vi "2011 Vision.vi"() -> ()   [LabVIEW 2013]
doc: "This example shows how to use color threshold, filtering, and particle analysis to locate reflective tape."
uses:
  Gridded Particles.ctl
  <vilib>/vision/NI_Vision_Development_Module.lvlib
panel:
  in  "stop":bool
  out "Annotated":T1(plugin-control)
  out "Threshold":T1(plugin-control)
  out "Original":T1(plugin-control)
  in  "Files":i32(listbox)
  in  "Filter":bool
  out "Columns":T2
  in  "Luma Range":cluster{"Lower value":i32, "Upper value":i32}={"Lower value"=91, "Upper value"=220}
  in  "Sat Range":cluster{"Lower value":i32, "Upper value":i32}={"Lower value"=50, "Upper value"=221}
  in  "Hue Range":cluster{"Lower value":i32, "Upper value":i32}={"Lower value"=234, "Upper value"=14}
  out "Histogram Xs":T3(graph)
  out "Particle Measurements (pixels)":dbl[][](array[numeric])
  in  "Selection Values":T5(array[cluster])=[{"Measurement Parameter"=35, "Range Lower Value"=5.0, "Range Upper Value"=300.0, "Range"=FALSE, "Measurement Type"=FALSE}] {"Measurement Parameter" items=["Center of Mass X", "Center of Mass Y", "First Pixel X", "First Pixel Y", "Bounding Rect Left", "Bounding Rect Top", "Bounding Rect Right", "Bounding Rect Bottom", "Max Feret Diameter Start X", "Max Feret Diameter Start Y", "Max Feret Diameter End X", "Max Feret Diameter End Y", "Max Horiz. Segment Length Left", "Max Horiz. Segment Length Right", "Max Horiz. Segment Length Row", "-", "Bounding Rect Width", "Bounding Rect Height", "Bounding Rect Diagonal", "Perimeter", "Convex Hull Perimeter", "Holes' Perimeter", "Max Feret Diameter", "Equivalent Ellipse Major Axis", "Equivalent Ellipse Minor Axis", "Equivalent Ellipse Minor Axis (Feret)", "Equivalent Rect Long Side", "Equivalent Rect Short Side", "Equivalent Rect Diagonal", "Equivalent Rect Short Side (Feret)", "Average Horiz. Segment Length", "Average Vert. Segment Length", "Hydraulic Radius", "Waddel Disk Diameter", "-", "Area", "Holes' Area", "Particle & Holes' Area", "Convex Hull Area", "Image Area", "-", "Number of Holes", "Number of Horiz. Segments", "Number of Vert. Segments", "-", "Orientation", "Max Feret Diameter Orientation", "-", "% Area/Image Area", "% Area/(Particle & Holes' Area)", "Ratio of Equivalent Ellipse Axes", "Ratio of Equivalent Rect Sides", "-", "Elongation Factor", "Compactness Factor", "Heywood Circularity Factor", "Type Factor", "-", "Sum X", "Sum Y", "Sum XX", "Sum XY", "Sum YY", "Sum XXX", "Sum XXY", "Sum XYY", "Sum YYY", "-", "Moment of Inertia XX", "Moment of Inertia XY", "Moment of Inertia YY", "Moment of Inertia XXX", "Moment of Inertia XXY", "Moment of Inertia XYY", "Moment of Inertia YYY", "Norm. Moment of Inertia XX", "Norm. Moment of Inertia XY", "Norm. Moment of Inertia YY", "Norm. Moment of Inertia XXX", "Norm. Moment of Inertia XXY", "Norm. Moment of Inertia XYY", "Norm. Moment of Inertia YYY", "Hu Moment 1", "Hu Moment 2", "Hu Moment 3", "Hu Moment 4", "Hu Moment 5", "Hu Moment 6", "Hu Moment 7"]}
  out "Particles post filter":i32
  # "1. Run the VI.\nSelect a folder containing images.\nUntil you abort, you can select an image\nin the list to process."
  # "2. Choose a color range to threshold.\nUse Hue, Saturation, and Luminance ranges. (0-255)\nNote that Red hue is near zero and it may be useful\nto reverse upper/lower to wrap around."
  # "3. Optionally filter using size or other measurements."
  # "4. Histogram indicates where poles are most likely found.\nImage is annotated with green squares around poles.\nParticle measurements can be examined further based on\nshape, size, grouping, location, etc. Columns describes\nthe three most likely columns.\n\nUse the toolbar Stop button to abort."
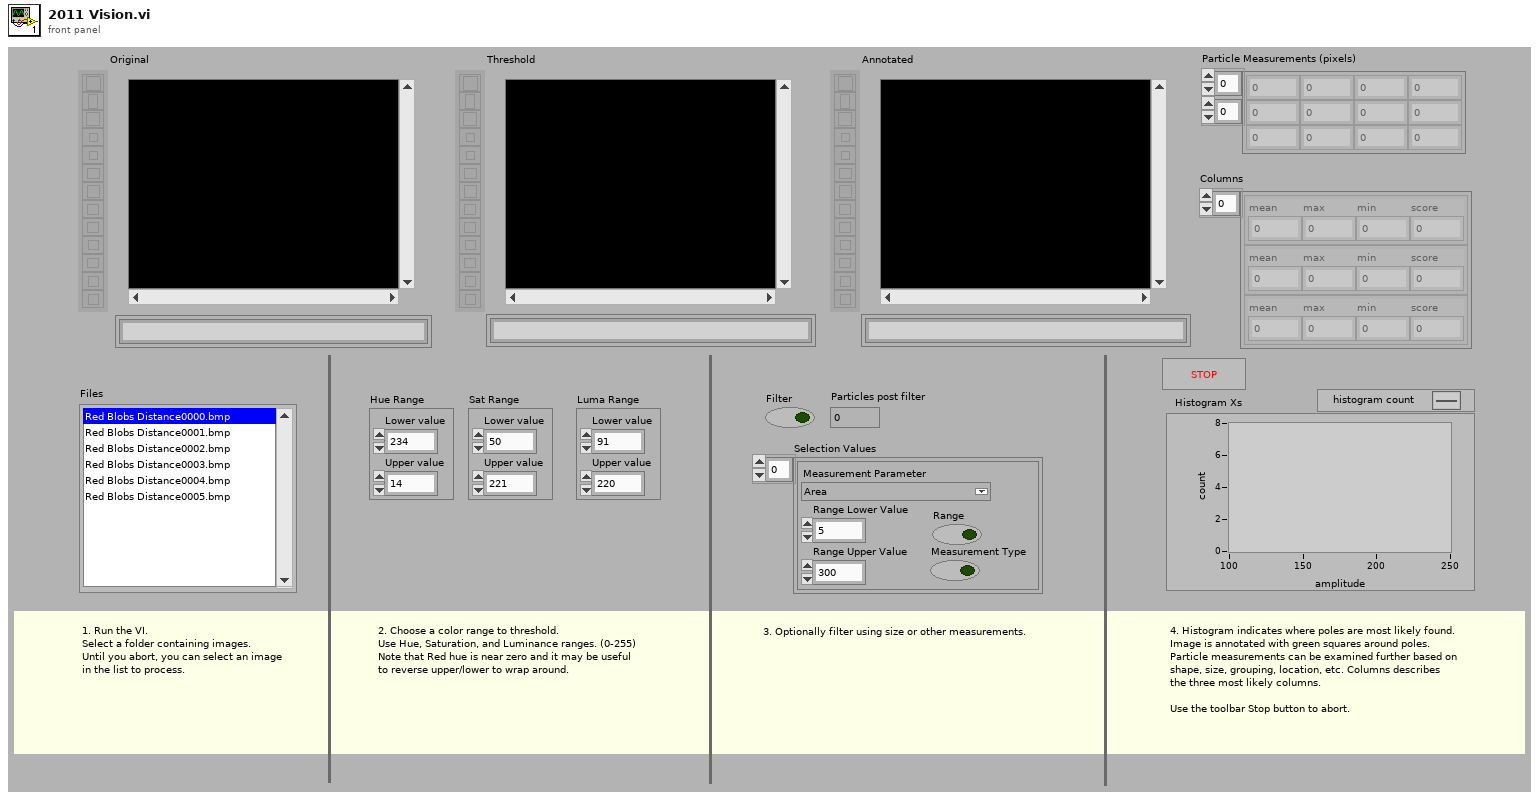
[diagram p1: front panel]
types:
  T1 = typedef "IMAQ Image.ctl" = refnum<image>
  T2 = typedef "Gridded Particles.ctl" = cluster{"mean":dbl, "max":dbl, "min":dbl, "score":dbl}[]
  T3 = cluster{"X Values":dbl[], "Histogram: h(x)":i32[]}
  T4 = typedef "Particle Parameters" = i32
  T5 = cluster{"Measurement Parameter":T4, "Range Lower Value":dbl, "Range Upper Value":dbl, "Range":bool, "Measurement Type":bool}[]
  T6 = typedef "Image Type" = u32
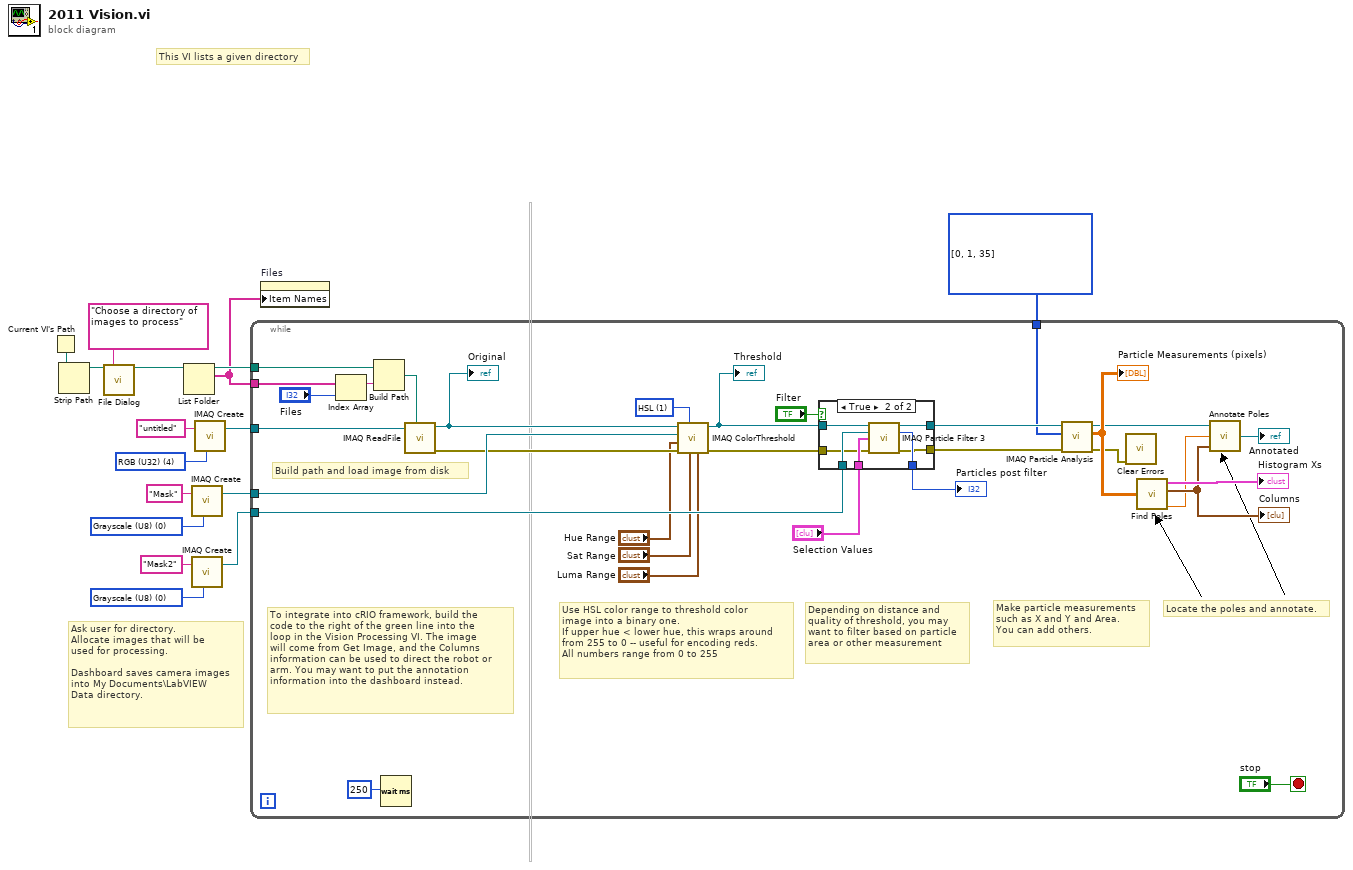
[diagram p0: block diagram]
diagram:
  w4 = T4[] [0, 1, 35] items=["Center of Mass X", "Center of Mass Y", "First Pixel X", "First Pixel Y", "Bounding Rect Left", "Bounding Rect Top", "Bounding Rect Right", "Bounding Rect Bottom", "Max Feret Diameter Start X", "Max Feret Diameter Start Y", "Max Feret Diameter End X", "Max Feret Diameter End Y", "Max Horiz. Segment Length Left", "Max Horiz. Segment Length Right", "Max Horiz. Segment Length Row", "-", "Bounding Rect Width", "Bounding Rect Height", "Bounding Rect Diagonal", "Perimeter", "Convex Hull Perimeter", "Holes' Perimeter", "Max Feret Diameter", "Equivalent Ellipse Major Axis", "Equivalent Ellipse Minor Axis", "Equivalent Ellipse Minor Axis (Feret)", "Equivalent Rect Long Side", "Equivalent Rect Short Side", "Equivalent Rect Diagonal", "Equivalent Rect Short Side (Feret)", "Average Horiz. Segment Length", "Average Vert. Segment Length", "Hydraulic Radius", "Waddel Disk Diameter", "-", "Area", "Holes' Area", "Particle & Holes' Area", "Convex Hull Area", "Image Area", "-", "Number of Holes", "Number of Horiz. Segments", "Number of Vert. Segments", "-", "Orientation", "Max Feret Diameter Orientation", "-", "% Area/Image Area", "% Area/(Particle & Holes' Area)", "Ratio of Equivalent Ellipse Axes", "Ratio of Equivalent Rect Sides", "-", "Elongation Factor", "Compactness Factor", "Heywood Circularity Factor", "Type Factor", "-", "Sum X", "Sum Y", "Sum XX", "Sum XY", "Sum YY", "Sum XXX", "Sum XXY", "Sum XYY", "Sum YYY", "-", "Moment of Inertia XX", "Moment of Inertia XY", "Moment of Inertia YY", "Moment of Inertia XXX", "Moment of Inertia XXY", "Moment of Inertia XYY", "Moment of Inertia YYY", "Norm. Moment of Inertia XX", "Norm. Moment of Inertia XY", "Norm. Moment of Inertia YY", "Norm. Moment of Inertia XXX", "Norm. Moment of Inertia XXY", "Norm. Moment of Inertia XYY", "Norm. Moment of Inertia YYY", "Hu Moment 1", "Hu Moment 2", "Hu Moment 3", "Hu Moment 4", "Hu Moment 5", "Hu Moment 6", "Hu Moment 7"] ("Pixel Measurements")
  w8 = T6 0 items=["Grayscale (U8)", "Grayscale (I16)", "Grayscale (SGL)", "Complex (CSG)", "RGB (U32)", "HSL (U32)", "RGB (U64)", "Grayscale (U16)"] ("Image Type")
  w12 = T6 0 items=["Grayscale (U8)", "Grayscale (I16)", "Grayscale (SGL)", "Complex (CSG)", "RGB (U32)", "HSL (U32)", "RGB (U64)", "Grayscale (U16)"] ("Image Type")
  w15 = T6 4 items=["Grayscale (U8)", "Grayscale (I16)", "Grayscale (SGL)", "Complex (CSG)", "RGB (U32)", "HSL (U32)", "RGB (U64)", "Grayscale (U16)"] ("Image Type")
  # "Ask user for directory.\nAllocate images that will be\nused for processing.\n\nDashboard saves camera images\ninto My Documents\\LabVIEW\nData directory."
  # "This VI lists a given directory"
  n1 = Current VI's Path() -> (path=w1:path)
  n2 = Strip Path(path=w1) -> (stripped path=w2:path)  [unwired: 1 out]
  n3 = call "File Dialog"("start path"=w2, "prompt"="Choose a directory of images to process") -> ("selected path"=w5:path)  [unwired: 5 in, 8 out]
  n4 = List Folder(path=w5) -> (path out=w13:path, filenames=w6:string[])  [unwired: 1 in, 4 out]
  n5 = call "IMAQ Create"("Image Name"="Mask", "Image Type"=w12) -> ("New Image"=w10:T1)  [unwired: 2 in, 2 out]
  n6 = call "IMAQ Create"("Image Name"="Mask2", "Image Type"=w8) -> ("New Image"=w7:T1)  [unwired: 2 in, 2 out]
  n7 = call "IMAQ Create"("Image Name"="untitled", "Image Type"=w15) -> ("New Image"=w14:T1)  [unwired: 2 in, 2 out]
  n8 = while {
    tunnel: w14 -> [w47]
    tunnel: w13 -> [w46]
    tunnel: w6 -> [w45]
    tunnel: w10 -> [w44]
    tunnel: w7 -> [w43]
    tunnel: w4 -> [w19]
    stop <- "stop" stop-if-true
    w22 = u16 1 items=["RGB", "HSL", "HSV", "HSI"] ("Color Mode")
    # "Locate the poles and annotate."
    # "To integrate into cRIO framework, build the\ncode to the right of the green line into the\nloop in the Vision Processing VI. The image\nwill come from Get Image, and the Columns\ninformation can be used to direct the robot or\narm. You may want to put the annotation\ninformation into the dashboard instead."
    # "Make particle measurements\nsuch as X and Y and Area.\nYou can add others."
    # "Depending on distance and\nquality of threshold, you may\nwant to filter based on particle\narea or other measurement"
    # "Use HSL color range to threshold color\nimage into a binary one.\nIf upper hue < lower hue, this wraps around\nfrom 255 to 0 -- useful for encoding reds.\nAll numbers range from 0 to 255"
    # "Build path and load image from disk"
    n9 = Index Array(array=w45, index="Files") -> (element=w33:string)
    n10 = Build Path(base path=w46, name or relative path=w33) -> (appended path=w40:path)
    n11 = Wait (ms)(milliseconds to wait=u32 250) -> ()  [unwired: 1 out]
    n12 = call "IMAQ ReadFile"("File Path"=w40, "Image"=w47) -> ("error out"=w36:errorcluster, "Image Out"=w23:T1)  [unwired: 3 in, 5 out]
    "Original" <- w23
    n13 = call "IMAQ ColorThreshold"("Blue or Luma or Val or Inten Range"="Luma Range", "Green or Sat Range"="Sat Range", "Color Mode"=w22, "error in (no error)"=w36, "Red or Hue Range"="Hue Range", "Image Dst"=w44, "Image Src"=w23) -> ("error out"=w35:errorcluster, "Image Dst Out"=w39:T1)  [unwired: 1 in, 2 out]
    "Threshold" <- w39
    n14 = case shown="True" "Filter" {
      tunnel: "Selection Values" -> [_ w56]
      tunnel: w43 -> [_ w55]
      tunnel: w39 -> [w49 w54]
      tunnel: [_ w53] -> w38
      tunnel: [w49 w52] -> w37
      tunnel: w35 -> [w48 w51]
      tunnel: [w48 w50] -> w27
      frame False {
      }
      frame True {
        n15 = call "IMAQ Particle Filter 3"("Image Src"=w54, "Image Dst"=w55, "Selection Values"=w56, "error in (no error)"=w51) -> ("Image Dst Out"=w52:T1, "Number of Particles"=w53:i32, "error out"=w50:errorcluster)  [unwired: 5 in, 4 out]
      }
    }
    "Particles post filter" <- w38
    n16 = call "IMAQ Particle Analysis"("error in (no error)"=w27, "Pixel Measurements"=w19, "Image"=w37) -> ("error out"=w20:errorcluster, "Particle Measurements (Pixels)"=w29:dbl[][], "Image Out (duplicate)"=w26:T1)  [unwired: 2 in, 4 out]
    "Particle Measurements (pixels)" <- w29
    n17 = call <vilib>:"Clear Errors.vi"("error in (no error)"=w20) -> ()  [unwired: 7 out]
    n18 = call "Find Poles.vi"("Particle Measurements"=w29) -> ("Histogram Particle Xs"=→"Histogram Xs":T3, "Grouped Particles"=w24:T2, "Spacing"=w18:dbl)  [unwired: 1 out]
    "Columns" <- w24
    n19 = call "Annotate Poles.vi"("Column Data"=w24, "Spacing"=w18, "Image In"=w26) -> ("Image Out"=→"Annotated":T1)
  }
  n20 = property on="Files" class="LstBox (strict)"("Item Names"=w6) -> ()  [unwired: 2 in, 2 out]
